vi "Open File.vi"(8 "error in (no error)":errorcluster, 11 "appended path":path) -> (0 "error out":errorcluster)   [LabVIEW 2019, in "Personalities Tool.lvlib"]
doc: "This VI opens a file in the command line"
uses:
  Personalities Tool.lvlib
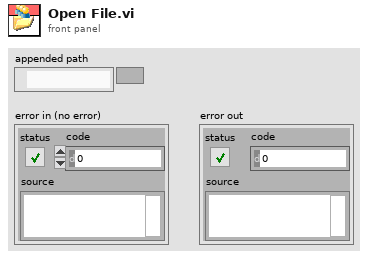
[diagram p1: front panel]
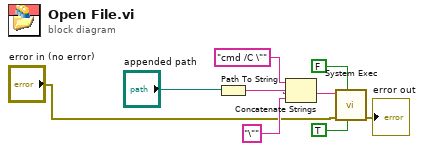
[diagram p0: block diagram]
diagram:
  n1 = Path To String(path="appended path") -> (string=w9:string)
  n2 = Concatenate Strings("cmd /C \"" ("string"), w9, "\"" ("string")) -> (w4:string)
  n3 = call <vilib>:"System Exec.vi"("run minimized? (F)"=TRUE, "wait until completion? (T)"=FALSE, "error in (no error)"="error in (no error)", "command line"=w4) -> ("error out"=→"error out":errorcluster)  [unwired: 4 in, 3 out]
